vi "Process Factory State.vi"(8 "error in (no error)":errorcluster, 11 "Network Session Handler in":refnum<class "Network Session Handler.lvclass">) -> (0 "error out":errorcluster, 3 "Network Session Handler out":refnum<class "Network Session Handler.lvclass">, 4 "Loop Timeout":i32)   [LabVIEW 2017, in "Network Interface.lvlib" / "Network Session Handler.lvclass"]
uses:
  <vilib>/gpm_packages/@cs/Network-sink/Source/Network Interface/Network Session Handler/Network Session Handler.lvclass
  <vilib>/gpm_packages/@cs/Network-sink/Source/Network Interface/Network Session Handler/Network Session Handler.lvclass/Network Session Handler.ctl
  <vilib>/gpm_packages/@cs/event-logger/Source/Composed Log/Types/Log Level.ctl
  <vilib>/gpm_packages/@cs/event-logger/Source/Composed Log/LoggerReference/LoggerReference.lvclass/LoggerReference.ctl
  <vilib>/gpm_packages/@cs/event-logger/Source/Composed Log/LoggerReference/Log.vi
  <vilib>/gpm_packages/@cs/event-logger/Source/Composed Log/LoggerReference/Get Valid Event Time.vi
  <vilib>/gpm_packages/@cs/event-logger/Source/Composed Log/LoggerReference/Remove Stale Logs.vi
  <vilib>/gpm_packages/@cs/event-logger/Source/Composed Log/Composed Log.lvlib
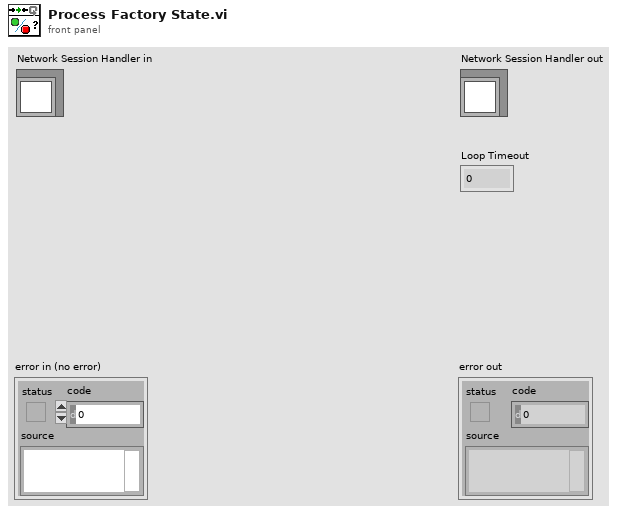
[diagram p1: front panel]
types:
  T1 = typedef "Composed Log.lvlib/Log Level.ctl" = enum16{"Debug", "Info", "Warning", "Error", "Critical"}
  T2 = typedef "Network Interface.lvlib/Network Session Handler.lvclass/Connection Handler.ctl" = cluster{"ID":string, "Handler Queue":refnum<class "Message Queue.lvclass">}
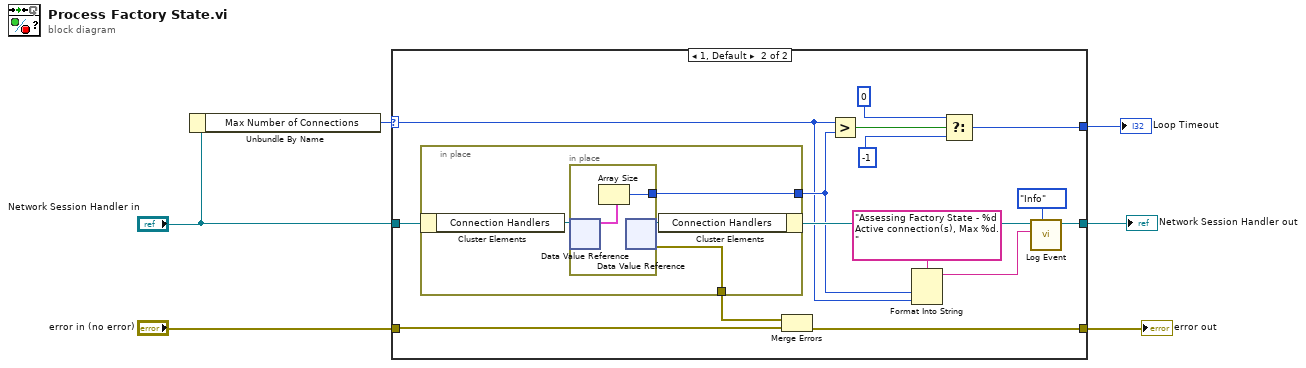
[diagram p0: block diagram]
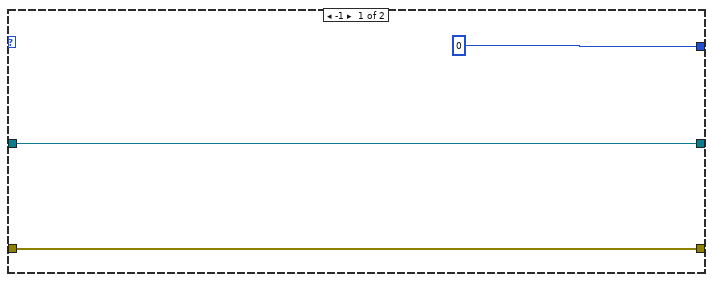
[diagram p2: hidden frame]
diagram:
  n1 = Unbundle By Name("Network Session Handler in") -> ("Max Number of Connections"=w4:i32)
  n2 = case shown="1, Default" w4 {
    selector: w4 -> [_ w11]
    tunnel: [w9 w14] -> w6
    tunnel: "Network Session Handler in" -> [w9 w20]
    tunnel: "error in (no error)" -> [w8 w19]
    tunnel: [w8 w17] -> w3
    tunnel: [0 ("f") w21] -> w2
    frame -1 {
    }
    frame 1, Default {
      n3 = in-place {
        in-place-border: [w26] -> w12
        in-place-border: [w25] -> w18
        n4 = in-place-cluster #1(w20) -> ("Connection Handlers"=w28:refnum<data-value>)
        n5 = in-place {
          in-place-border: [w29] -> w26
          n6 = in-place-dvr #2(w28) -> (w30:T2[])  [unwired: 1 out]
          n7 = Array Size(array=w30) -> (size(s)=w29:i32)
          n8 = in-place-dvr #2() -> (w27:refnum<data-value>, w25:errorcluster)  [unwired: 1 in]
        }
        n9 = in-place-cluster #1("Connection Handlers"=w27) -> (w15:refnum<class "Network Session Handler.lvclass">)
      }
      n10 = Merge Errors(w18, w19) -> (w17:errorcluster)
      n11 = Greater?(x=w11, y=w12) -> (0:w24:bool)
      n12 = Format Into String(format string="Assessing Factory State - %d Active connection(s), Max %d." ("Event"), w12, w11) -> (resulting string=w10:string)  [unwired: 2 in, 1 out]
      n13 = Select(t=0, s=w24, f=-1) -> (s? t:f=w21:i32)
      n14 = call <vilib>:"Log Event.vi"("Event Level"=Log_Level."Info", "Event"=w10, "Network Session Handler in"=w15) -> ("Network Session Handler out"=w14:refnum<class "Network Session Handler.lvclass">)  [unwired: 7 in, 1 out]
    }
  }
  "error out" <- w3
  "Network Session Handler out" <- w6
  "Loop Timeout" <- w2
